vi "Replace Or Add Robots.vi"(10 "Robots New":T1[](array[typedef]) {"height" format="%+4.3f"; "pixel_y" format="%+4.3f"; "pixel_x" format="%+4.3f"; "orientation" format="%+4.3f"; "y" format="%+4.3f"; "confidence" format="%4.3f"; "x" format="%+4.3f"}, 11 "Robots Old":T1[](array[typedef]) {"height" format="%+4.3f"; "pixel_y" format="%+4.3f"; "pixel_x" format="%+4.3f"; "orientation" format="%+4.3f"; "y" format="%+4.3f"; "confidence" format="%4.3f"; "x" format="%+4.3f"}) -> (3 "Robots New Out":T1[](array[typedef]) {"height" format="%+4.3f"; "pixel_y" format="%+4.3f"; "pixel_x" format="%+4.3f"; "orientation" format="%+4.3f"; "y" format="%+4.3f"; "confidence" format="%4.3f"; "x" format="%+4.3f"})   [LabVIEW 2018]
uses:
  git/SSLView/SSL Detection Robot.ctl
  <vilib>/Analysis/Matrix/Datatypes/RealMatrix.ctl
  <vilib>/Analysis/Matrix/NI_Matrix.lvlib
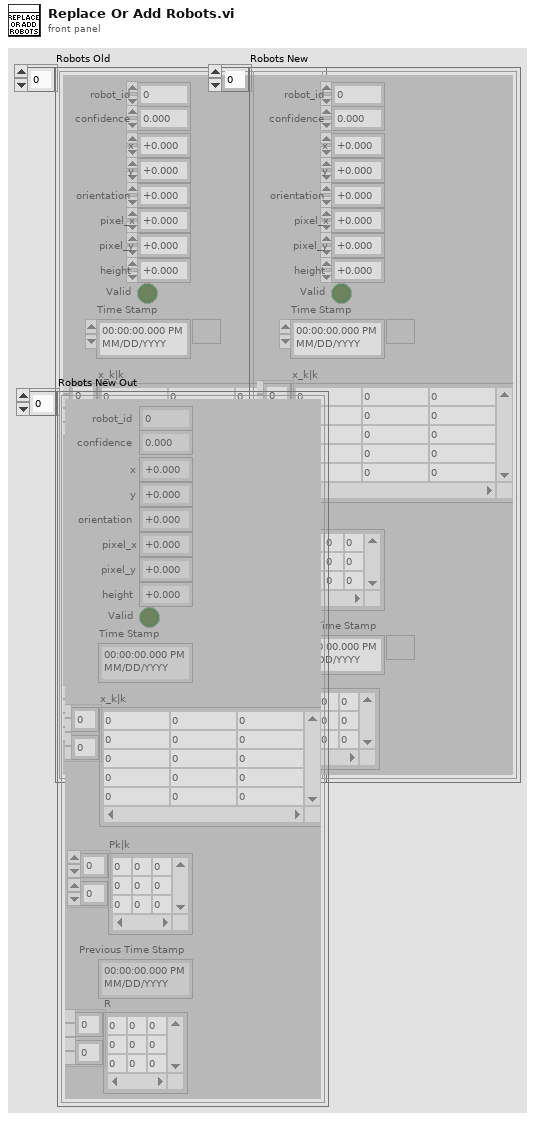
[diagram p1: front panel]
types:
  T1 = typedef "SSL Detection Robot.ctl" = cluster{"x":sgl, "robot_id":u32, "confidence":sgl, "y":sgl, "orientation":sgl, "pixel_x":sgl, "pixel_y":sgl, "height":sgl, "Valid":bool, "Time Stamp":timestamp, "x_k|k":T2, "Pk|k":T2, "Previous Time Stamp":timestamp, "R":T2}
  T2 = typedef "NI_Matrix.lvlib/RealMatrix.ctl" = dbl[][]
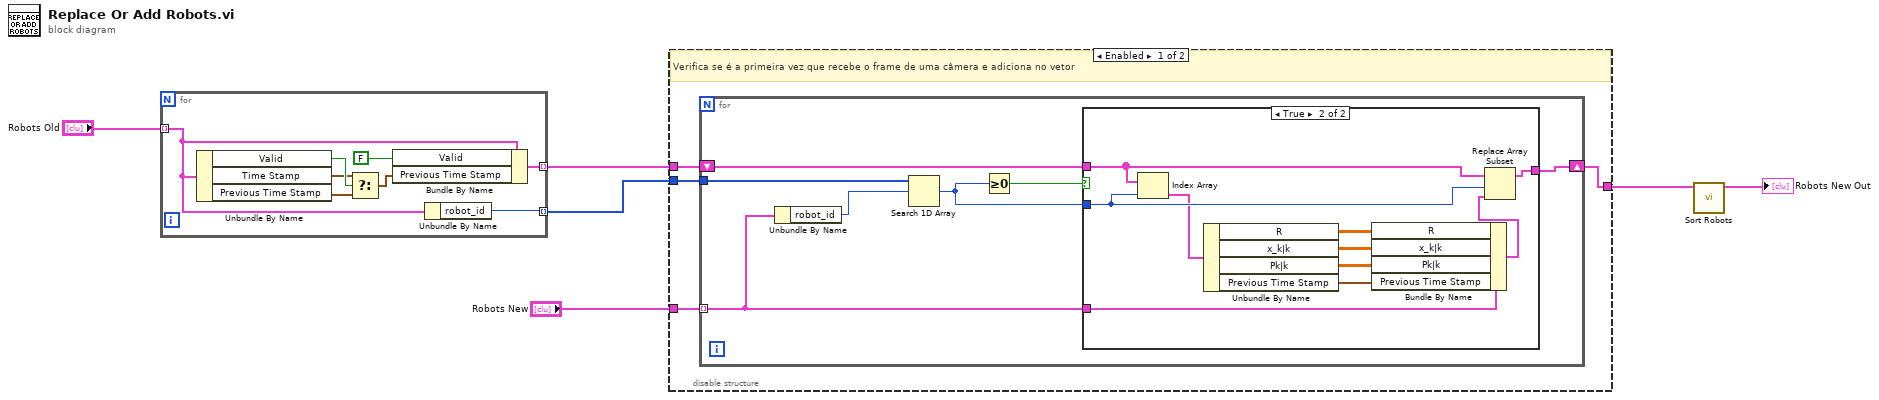
[diagram p0: block diagram]
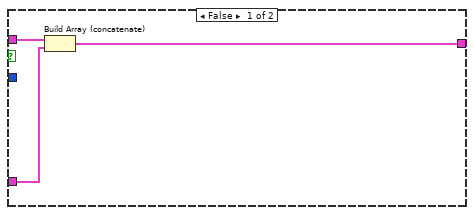
[diagram p2: hidden frame]
diagram:
  n1 = for {
    tunnel: "Robots Old" -> [w11] mode=indexing
    tunnel: [w14] -> w5 mode=indexing
    tunnel: [w12] -> w3 mode=indexing
    n2 = Unbundle By Name(w11) -> ("Valid"=w10:bool, "Time Stamp"=w9:timestamp, "Previous Time Stamp"=w7:timestamp)
    n3 = Select(t=w9, s=w10, f=w7) -> (s? t:f=w8:timestamp)
    n4 = Bundle By Name(cluster=w11, "Valid"=FALSE, "Previous Time Stamp"=w8) -> (w12:T1)
    n5 = Unbundle By Name(w11) -> ("robot_id"=w14:u32)
  }
  n6 = disable-structure "Diagram Disable Structure" shown="Enabled" {
    disable-tunnel: w3 -> [w18 _]
    disable-tunnel: "Robots New" -> [w17 _]
    disable-tunnel: [w16 _] -> w2
    disable-tunnel: w5 -> [w15 _]
    frame Enabled {
      # "Verifica se é a primeira vez que recebe o frame de uma câmera e adiciona no vetor"
      n7 = for {
        tunnel: w17 -> [w22] mode=indexing
        tunnel: w15 -> [w23]
        shift-right: [w24] -> w16
        shift-left: w18 -> [w25]
        n8 = Unbundle By Name(w22) -> ("robot_id"=w21:u32)
        n9 = Search 1D Array(1D array=w23, element=w21) -> (index of element=w19:i32)  [unwired: 1 in]
        n10 = Greater Or Equal To 0?(x=w19) -> (x >= 0?=w20:bool)
        n11 = case shown="True" w20 {
          tunnel: w25 -> [w28 w37]
          tunnel: w22 -> [w26 w34]
          tunnel: [w27 w38] -> w24
          tunnel: w19 -> [_ w36]
          frame False {
            n12 = Build Array (concatenate)(w28, w26) -> (w27:T1[])
          }
          frame True {
            n13 = Index Array(array=w37, index=w36) -> (element=w35:T1)
            n14 = Unbundle By Name(w35) -> ("R"=w29:T2, "x_k|k"=w32:T2, "Pk|k"=w31:T2, "Previous Time Stamp"=w30:timestamp)
            n15 = Bundle By Name(cluster=w34, "R"=w29, "x_k|k"=w32, "Pk|k"=w31, "Previous Time Stamp"=w30) -> (w33:T1)
            n16 = Replace Array Subset(array=w37, new element=w33, index=w36) -> (w38:T1[])
          }
        }
      }
    }
    frame Disabled {
    }
  }
  n17 = call "Sort Robots.vi"("robots_blue"=w2) -> ("Array"=→"Robots New Out":T1[])  [unwired: 10 in]
